vi "Set WIFI Password.vi"(8 "Error In":errorcluster, 10 "Password":string, 11 "LINX Device Config":T1) -> (0 "Error Out":errorcluster, 3 "LINX Device Config":T1)   [LabVIEW 2013, in "LVH-LINX.lvlib" / "Device.lvlib"]
doc: "Set the LINX device's WIFI SSID."
uses:
  Device.lvlib
  Type Defs/LINX Device Config.ctl
  Type Defs/Interface.ctl
  Type Defs/TCP Config.ctl
  Type Defs/Device Family.ctl
  Type Defs/Channels.ctl
  Type Defs/Error Type.ctl
  LVH-LINX.lvlib
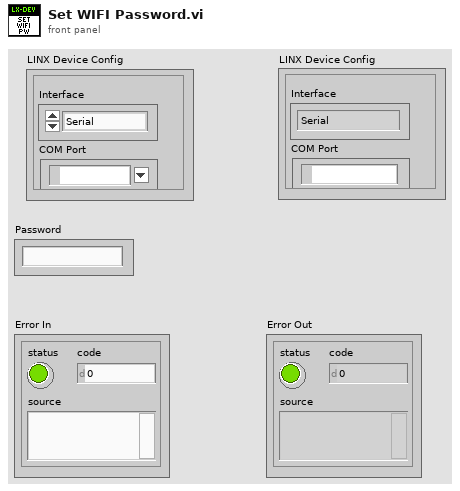
[diagram p1: front panel]
types:
  T1 = typedef "LVH-LINX.lvlib/Device.lvlib/LINX Device Config.ctl" = cluster{"Interface":T2, "COM Port":refnum<visa-resource-name>, "TCP Configuration":T3, "Device Family":T4, "Device ID":u8, "Device Name":string, "TCP Ref":refnum<k5>, "Channels":T5}
  T2 = typedef "LVH-LINX.lvlib/Interface.ctl" = enum16{"Serial", "TCP"}
  T3 = typedef "LVH-LINX.lvlib/Device.lvlib/TCP Config.ctl" = cluster{"IP Address":string, "Port":u16}
  T4 = typedef "LVH-LINX.lvlib/Device Family.ctl" = enum8{"National Instruments", "Digilent", "Arduino"}
  T5 = typedef "LVH-LINX.lvlib/Channels.ctl" = cluster{"DI Channels":u8[], "DO Channels":u8[], "AI":u8[], "AO":u8[], "PWM":u8[], "QE":u8[], "UART":u8[], "I2C 2":u8[], "SPI":u8[], "CAN":u8[], "AI Ref (V)":dbl, "AO Resolution (Bits)":u8, "AO Ref (V)":dbl}
  T6 = typedef "LVH-LINX.lvlib/Error Type.ctl" = enum16{"Unknown", "Timeout", "Corrupt Return Packet", "Unable To Connect", "Command Not Supported", "Channel DNE", "Invalid COM Config", "Firmware Version Mismatch"}
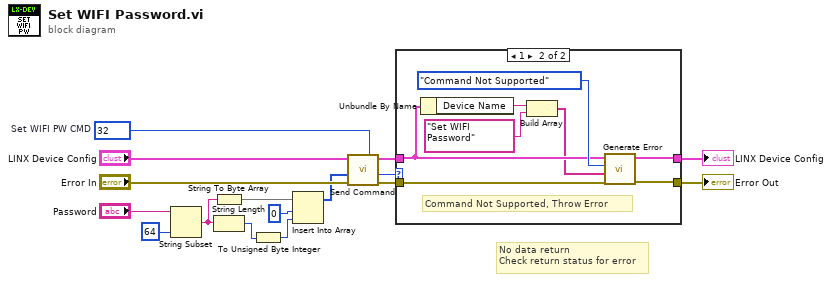
[diagram p0: block diagram]
diagram:
  w15 = u16 32  # Set WIFI PW CMD
  # "No data return\nCheck return status for error"
  n1 = String Subset(string="Password", length (rest)=64 ("length (rest)")) -> (substring=w5:string)  [unwired: 1 in]
  n2 = String To Byte Array(string=w5) -> (unsigned byte array=w4:u8[])
  n3 = String Length(string=w5) -> (length=w8:i32)
  n4 = To Unsigned Byte Integer(number=w8) -> (unsigned 8bit integer=w3:u8)
  n5 = Insert Into Array(array=w4, index=0, new element=w3) -> (w1:u8[])
  n6 = call "Send Command.vi"("Error In"="Error In", "ARGS"=w1, "CMD"=w15, "LINX Device Config"="LINX Device Config") -> ("Error Out"=w10:errorcluster, "Status"=w9:u8, "LINX Device Config"=w12:T1)  [unwired: 4 in, 1 out]
  n7 = case shown="1" w9 {
    tunnel: [w17 w24] -> w13
    tunnel: w12 -> [w17 w20]
    tunnel: [w18 w25] -> w11
    tunnel: w10 -> [w18 w26]
    frame 0, Default {
      # "Status OK, Process Data"
    }
    frame 1 {
      # "Command Not Supported, Throw Error"
      n8 = Unbundle By Name(w20) -> ("Device Name"=w21:string)
      n9 = Build Array(w21, "Set WIFI Password") -> (w19:string[])
      n10 = call "Generate Error.vi"("Error In"=w26, "Arguments"=w19, "Error Type"=Error_Type."Command Not Supported", "LINX Device Config"=w20) -> ("Error Out"=w25:errorcluster, "LINX Device Config"=w24:T1)  [unwired: 6 in]
    }
  }
  "Error Out" <- w11
  "LINX Device Config" <- w13
